vi "Database.Cache.Reload.vi"(7 "Idx":i32, 8 "error in":errorcluster) -> (0 "error out":errorcluster)   [LabVIEW 2016]
doc: "Connect to database\n\nWabco 2017 All right reserved\nAuthor: maciej.szupienko@wabco-auto.com"
uses:
  Cache/Cache.TestSteps.Fglb.Action.ctl
  Cache/Cache.TestSteps.Fglb.ResultData.ctl
  ProdaNG/Controls/ProdaNG.ProcessResult.ctl
  ProdaNG/Controls/ProdaNG.ProcessStepResult.ctl
  ProdaNG/Controls/ProdaNG.TestStepResult.ctl
  ProdaNG/Controls/ProdaNG.TestValueResult.ctl
  Database.Global.vi
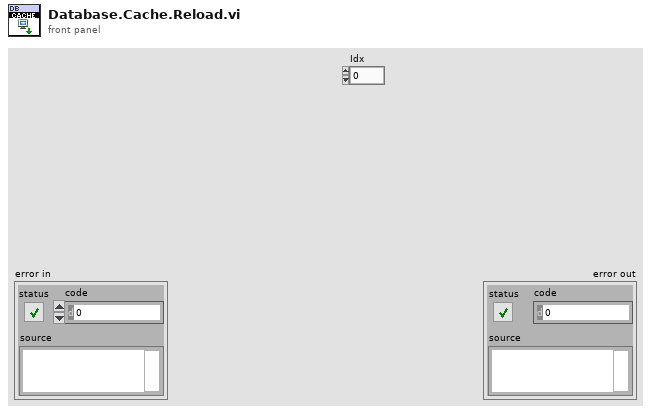
[diagram p1: front panel]
types:
  T1 = typedef "Cache.TestSteps.Fglb.ResultData.ctl" = cluster{"File":path, "Ref":string, "Serial":string, "Pr":T2, "PSr":T3, "TSr":cluster{"TSr":T4, "TVr":T5[]}[]}
  T2 = typedef "ProdaNG.ProcessResult.ctl" = cluster{"c_id":string, "productId":string, "processId":i32, "statusId":i32, "startTime":string, "endTime":string}
  T3 = typedef "ProdaNG.ProcessStepResult.ctl" = cluster{"c_id":string, "processResultId":string, "processStepId":i32, "statusId":i32, "operatorId":i32, "startTime":string, "endTime":string}
  T4 = typedef "ProdaNG.TestStepResult.ctl" = cluster{"c_id":string, "processStepResultId":string, "testStepId":i32, "statusId":i32}
  T5 = typedef "ProdaNG.TestValueResult.ctl" = cluster{"c_id":string, "testStepResultId":string, "testValueId":i32, "result":dbl, "statusId":i32, "contentId":string}
  T6 = typedef "Cache.TestSteps.Fglb.Action.ctl" = enum16{"init", "add", "get"}
  T7 = typedef "Cache.TestSteps.Fglb.TestData.ctl" = cluster{"Ref":string, "Desc":string, "P":T8, "PS":T9, "PP":T10[], "TS":cluster{"TS":T11, "TV":T12[], "TP":T13[]}[], "Units":T14[]}
  T8 = typedef "ProdaNG.Process.ctl" = cluster{"i_id":i32, "productionLineId":i32, "releaseId":i32, "contentId":string, "previewId":string, "mdReason":string, "mdUser":string, "mdTime":string, "description":string}
  T9 = typedef "ProdaNG.ProcessStep.ctl" = cluster{"i_id":i32, "processId":i32, "systemId":i32, "releaseId":i32, "processSequence":i32, "limitYellow":dbl, "limitRed":dbl, "mdReason":string, "mdUser":string, "mdTime":string, "filename":string, "transfer":string, "description":string}
  T10 = typedef "ProdaNG.ProcessStepParam.ctl" = cluster{"i_id":i32, "processStepId":i32, "unitId":i32, "contentId":string, "previewId":string, "value":dbl, "valueText":string, "paramSequence":i32, "history":i32, "mdReason":string, "mdUser":string, "mdTime":string, "description":string}
  T11 = typedef "ProdaNG.TestStep.ctl" = cluster{"i_id":i32, "processStepId":i32, "testSequence":i32, "testOrder":i32, "mdReason":string, "mdUser":string, "mdTime":string, "description":string}
  T12 = typedef "ProdaNG.TestValue.ctl" = cluster{"i_id":i32, "testStepId":i32, "releaseId":i32, "unitId":i32, "contentId":string, "previewId":string, "maximum":dbl, "minimum":dbl, "valueText":string, "testValueSequence":i32, "history":i32, "mdReason":string, "mdUser":string, "mdTime":string, "description":string}
  T13 = typedef "ProdaNG.TestStepParam.ctl" = cluster{"i_id":i32, "testStepId":i32, "unitId":i32, "contentId":string, "previewId":string, "value":dbl, "valueText":string, "paramSequence":i32, "history":i32, "mdReason":string, "mdUser":string, "mdTime":string, "description":string}
  T14 = typedef "ProdaNG.Unit.ctl" = cluster{"i_id":i32, "name":string, "mdReason":string, "mdUser":string, "mdTime":string, "description":string}
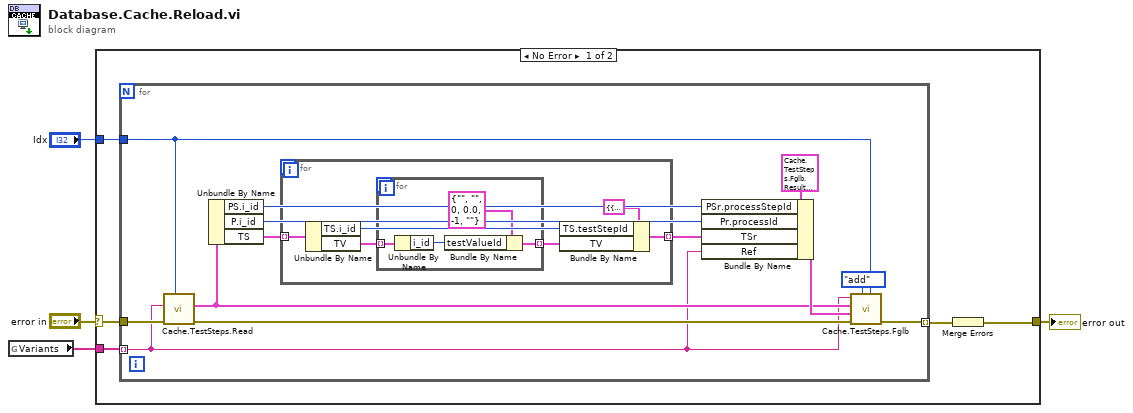
[diagram p0: block diagram]
diagram:
  n1 = global read "Database.Global.vi" "Variants"() -> (w1:string[])
  n2 = case shown="No Error" "error in" {
    selector: "error in" -> [w9 w33]
    tunnel: [w8 w33] -> w4
    tunnel: "Idx" -> [w7 _]
    tunnel: w1 -> [w5 _]
    frame No Error {
      n3 = for {
        tunnel: w5 -> [w10] mode=indexing
        tunnel: w9 -> [w22]
        tunnel: w7 -> [w17]
        tunnel: [w12] -> w6 mode=indexing
        n4 = call "Cache.TestSteps.Read.vi"("Idx"=w17, "error in (no error)"=w22, "Ref"=w10) -> ("error out"=w18:errorcluster, "TS in"=w11:T7)  [unwired: 7 in]
        n5 = Unbundle By Name(w11) -> ("PS.i_id"=w14:i32, "P.i_id"=w15:i32, "TS"=w21:cluster{"TS":T11, "TV":T12[], "TP":T13[]}[])
        n6 = for {
          tunnel: [w25] -> w13 mode=indexing
          tunnel: w21 -> [w24] mode=indexing
          n7 = Unbundle By Name(w24) -> ("TS.i_id"=w27:i32, "TV"=w23:T12[])
          n8 = for {
            tunnel: w23 -> [w32] mode=indexing
            tunnel: [w29] -> w28 mode=indexing
            n9 = Unbundle By Name(w32) -> ("i_id"=w31:i32)
            n10 = Bundle By Name(cluster=T5 {"c_id"="", "testStepResultId"="", "testValueId"=0, "result"=0.0, "statusId"=-1, "contentId"=""} ("TV"), "testValueId"=w31) -> (w29:T5)
          }
          n11 = Bundle By Name(cluster=cluster{"TS":T4, "TV":T5[]} {"TS"={"c_id"="", "processStepResultId"="", "testStepId"=0, "statusId"=-1}, "TV"=[]} ("Cluster"), "TS.testStepId"=w27, "TV"=w28) -> (w25:cluster{"TS":T4, "TV":T5[]})
        }
        n12 = Bundle By Name(cluster=T1 {"File"=path "", "Ref"="", "Serial"="", "Pr"={"c_id"="", "productId"="", "processId"=0, "statusId"=0, "startTime"="", "endTime"=""}, "PSr"={"c_id"="", "processResultId"="", "processStepId"=0, "statusId"=0, "operatorId"=0, "startTime"="", "endTime"=""}, "TSr"=[]} ("Result in"), "PSr.processStepId"=w14, "Pr.processId"=w15, "TSr"=w13, "Ref"=w10) -> (w19:T1)
        n13 = call "Cache.TestSteps.Fglb.vi"("SystemIdx"=w17, "Action (get)"=Cache.TestSteps.Fglb.Action."add", "error in (no error)"=w18, "Result in"=w19, "Test in"=w11, "Variant"=w10) -> ("error out"=w12:errorcluster)  [unwired: 2 in, 3 out]
      }
      n14 = Merge Errors(w6) -> (w8:errorcluster)
    }
    frame Error {
    }
  }
  "error out" <- w4
